vi "dvp Vi Get Quick Roi Sel Descr.vi"(9 "puCount":u32, 10 "puDefault":u32, 11 "handle":u32) -> (1 "puCount out":u32, 2 "puDefault out":u32, 3 "function return":u32(ring))   [LabVIEW 2018, in "LabViewDVPCamera.lvlib"]
doc: "LabviewDvp2Api dvpStatus dvpViGetQuickRoiSelDescr(\n dvpHandle handle, \n dvpUint32 *puDefault,\n dvpUint32 *puCount);"
uses:
  LabViewDVPCamera.lvlib
  LabViewDVPCamera/LabViewDVPCamera.dll
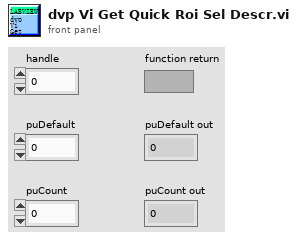
[diagram p1: front panel]
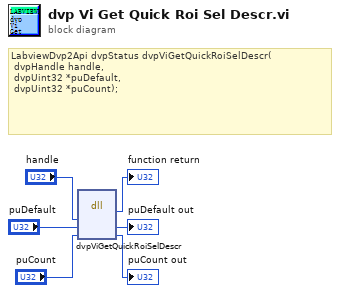
[diagram p0: block diagram]
diagram:
  # "LabviewDvp2Api dvpStatus dvpViGetQuickRoiSelDescr(\n\tdvpHandle handle, \n\tdvpUint32 *puDefault,\n\tdvpUint32 *puCount);"
  n1 = dll-call lib="C:/Program Files (x86)/DVP2 Labview cn 64/Sample/LabViewDVPCamera/LabViewDVPCamera.*" fn="dvpViGetQuickRoiSelDescr"("handle"="handle", "puDefault"="puDefault", "puCount"="puCount") -> (→"function return":u32, "puDefault"=→"puDefault out":u32, "puCount"=→"puCount out":u32)  [unwired: 4 in, 2 out]
